vi "sonde front panel.vi"() -> ()   [LabVIEW 2016]
uses:
  SDI-12/Sonde Vertical Graph.ctl
  Waterloo DAQ/controls/Vertical Chart.ctl
  activeXtest/activeXtest 2015 Folder/sample data row cluster.ctl
  activeXtest/activeXtest 2015 Folder/sonde cluster.ctl
  Groundwater header.ctl
  Waterloo DAQ/controls/MCC DAQ Setup.ctl
  Waterloo DAQ/controls/Aux Sensor.ctl
  KPRO_2016 subvis/Control 2.ctl
  KPRO_2016 subvis/Control 9.ctl
  KPRO_2016 subvis/Graph Controls 2.ctl
  KPRO_2016 subvis/Ik control.ctl
  KPRO_2016 subvis/Ion Slope Control 8.ctl
  KPRO_2016 subvis/Depth Control.ctl
  KPRO_2016 subvis/SS Control 7.ctl
  Waterloo DAQ/controls/Action Control 1.ctl
  <extravilib>/ChannelInstances/One Element Stream-t'Action Control 1.ctl'/Instantiate.vi
  <extravilib>/ChannelInstances/One Element Stream-t'Action Control 1.ctl'/Endpoint.vi
  <vilib>/ULx/Create Channel.llb/ULx Create Channel (AI-Voltage-Basic).vi
  <vilib>/ULx/Read.llb/ULx Read (Analog DBL 1Chan 1Samp).vi
  C:/Program Files (x86)/National Instruments/LabVIEW 2016/vi.lib/ULx/ULx_LV.dll
  <vilib>/Utility/NIReport.llb/NI_report.lvclass
  <vilib>/Utility/config.llb/NI_LVConfig.lvlib
  <extravilib>/ChannelInstances/One Element Stream-t'Action Control 1.ctl'.lvlib
panel:
  out "Feet of Stainless 2":i32
  out "Feet of\nStainless to be\nUsed (Count)":i32
  in  "SS In":i32
  in  "Record Continuous Samples":bool
  out "Current Time (s)":dbl
  in  "Sample Sheet Data Row Cluster 2":T1={"Head"=0.0, "Depth"=0.0, "comment string"="", "Sonde Data Cluster"={"Cumulative\nVolume"=100.0, "Specific\nConductance"=2.0, "Dissolved\nOxygen"=3.0, "pH"=4.0, "ORP"=5.0, "Temp"=26.0, "Salinity"=7.0}} {"Sonde Data Cluster"."Salinity" format="%_3g"; "Sonde Data Cluster"."Temp" format="%_2g"; "Sonde Data Cluster"."ORP" format="%_4g"; "Sonde Data Cluster"."pH" format="%_4g"; "Sonde Data Cluster"."Dissolved\nOxygen" format="%_4g"; "Sonde Data Cluster"."Specific\nConductance" format="%_4g"; "Sonde Data Cluster"."Cumulative\nVolume" format="%#_4g"}
  in  "stop":bool
  in  "Write Data to Spreadsheet":bool
  in  "Sample Not Collected":bool
  in  "Record Single Sample":bool
  in  "Tab Control":T3(tab)
  out "12V Voltage Monitor":dbl format="%_3f"
  out "Found Quanta Sonde Com Port":refnum<visa-resource-name>
  in  "Temporary Data Files Directory":path=path "D:/Cascade/Data/Raw Sonde Data"
  in  "Data File Directory":path=path "D:/Cascade/Data/Excel Reports"
  out "Quanta Sonde found?":bool
  in  "report file path":path=path "D:/Cascade/templates/Groundwater Profiling Log_empty_2.xlsx"
  in  "template file path":path=path "D:/Cascade/templates/Groundwater Profiling Log_empty_labview_template.xlsx"
  in  "Config File Path":path=path "D:/Cascade/Data/config files/DAQ Setup Config.ini"
  in  "Read Configuration File?":bool=TRUE
  out "H-4191 Adapter found":bool
  in  "Save Configuration File?":bool
  out "Sonde Communication Error Out":errorcluster
  in  "Search for Comm Ports?":bool=TRUE
  in  "USB Serial Port Manual Entry":refnum<visa-resource-name>="COM13"
  in  "MCC USB-DAQ Setup":T4={"Device Name in InstaCal"="Dev0", "Omega Pressure Sensor"={"DAQ Channel"=2.0, "Output Voltage Range"=1, "Enabled"=TRUE, "Description"="Uphole Pressure"}, "McMillian 102 Flowmeter"={"DAQ Channel"=11.0, "Output Voltage Range"=1, "Enabled"=TRUE, "Description"="Flow"}, "DHT Pressure Sensor"={"DAQ Channel"=3.0, "Output Voltage Range"=1, "Enabled"=TRUE, "Description"="Downhole Pressure"}, "Top String Pot"={"DAQ Channel"=0.0, "Output Voltage Range"=0, "Enabled"=TRUE, "Description"="Top String Pot"}, "String Pot Signal"={"DAQ Channel"=1.0, "Output Voltage Range"=0, "Enabled"=TRUE, "Description"="String Pot"}, "Aux Sensor 1"={"DAQ Channel"=5.0, "Output Voltage Range"=1, "Enabled"=FALSE, "Description"="Aux 1"}, "Aux Sensor 2"={"DAQ Channel"=6.0, "Output Voltage Range"=1, "Enabled"=FALSE, "Description"="Aux 2"}, "Aux Sensor 3"={"DAQ Channel"=7.0, "Output Voltage Range"=1, "Enabled"=TRUE, "Description"="Aux 3"}, "Voltage Monitor"={"DAQ Channel"=8.0, "Output Voltage Range"=0, "Enabled"=TRUE, "Description"="9V Monitor"}} {"Voltage Monitor"."Output Voltage Range" items=["+/-10 V Range", "+/-5 V Range", "+/-2.5V Range", "+/-1.25 V Range", "+/-0.625 V Range", "+/-0.3125 V Range", "+/-0.1562V Range", "+/-0.078125 V Range"]; "Aux Sensor 3"."Output Voltage Range" items=["+/-10 V Range", "+/-5 V Range", "+/-2.5V Range", "+/-1.25 V Range", "+/-0.625 V Range", "+/-0.3125 V Range", "+/-0.1562V Range", "+/-0.078125 V Range"]; "Aux Sensor 2"."Output Voltage Range" items=["+/-10 V Range", "+/-5 V Range", "+/-2.5V Range", "+/-1.25 V Range", "+/-0.625 V Range", "+/-0.3125 V Range", "+/-0.1562V Range", "+/-0.078125 V Range"]; "Aux Sensor 1"."Output Voltage Range" items=["+/-10 V Range", "+/-5 V Range", "+/-2.5V Range", "+/-1.25 V Range", "+/-0.625 V Range", "+/-0.3125 V Range", "+/-0.1562V Range", "+/-0.078125 V Range"]; "String Pot Signal"."Output Voltage Range" items=["+/-10 V Range", "+/-5 V Range", "+/-2.5V Range", "+/-1.25 V Range", "+/-0.625 V Range", "+/-0.3125 V Range", "+/-0.1562V Range", "+/-0.078125 V Range"]; "Top String Pot"."Output Voltage Range" items=["+/-10 V Range", "+/-5 V Range", "+/-2.5V Range", "+/-1.25 V Range", "+/-0.625 V Range", "+/-0.3125 V Range", "+/-0.1562V Range", "+/-0.078125 V Range"]; "DHT Pressure Sensor"."Output Voltage Range" items=["+/-10 V Range", "+/-5 V Range", "+/-2.5V Range", "+/-1.25 V Range", "+/-0.625 V Range", "+/-0.3125 V Range", "+/-0.1562V Range", "+/-0.078125 V Range"]; "McMillian 102 Flowmeter"."Output Voltage Range" items=["+/-10 V Range", "+/-5 V Range", "+/-2.5V Range", "+/-1.25 V Range", "+/-0.625 V Range", "+/-0.3125 V Range", "+/-0.1562V Range", "+/-0.078125 V Range"]; "Omega Pressure Sensor"."Output Voltage Range" items=["+/-10 V Range", "+/-5 V Range", "+/-2.5V Range", "+/-1.25 V Range", "+/-0.625 V Range", "+/-0.3125 V Range", "+/-0.1562V Range", "+/-0.078125 V Range"]}
  out "Rate":dbl=1000.0 caption="Sample Rate (Hz)"
  out "Number of Channels":u16
  in  "Channel Data Rate S/s":dbl=3720.0 format="%#_13g"
  out "Descriptions":string[](array[string])
  out "Raw Voltages":dbl[](array[numeric])
  out "9V Voltage Monitor":dbl
  in  "Record DAQ Raw Voltages":bool
  in  "Groundwater Header":T6
  out "Worksheet Names":string[](array[string])
  in  "Current Sheet":i32=1
  out "row max value":i32
  out "last occupied cell's name":string
  out "Current Sample Sheet":string="Sample 1"
  in  "Cluster":T7={"Profile ID"="WP-01", "Hole Id"="HOLE_001"}
  out "Sonde Data Array":string[][](array[string])
  out "Table Label":string="Data from Sample Sheet %d from Excel File"
  out "Sonde Data Display":T8
  out "Temperature":cluster{"Y":dbl[], "Y":dbl[]}[](graph)
  in  "Record Reason":bool
  in  "Select Reasons to Record Data":u16(ring) items=["Per Client Request", "Timed Out", "Sample stopped flowing", "Equipment Issue"]
  in  "Record Calibration Values":bool
  in  "Ion Offset":dbl format="%.2f"
  in  "Ion Slope":dbl=44.04 format="%.2f"
  in  "Pressure \nSlope":dbl=24.27199935913086 format="%.2f"
  in  "Flow Slope":dbl=37.99800109863281 format="%.2f"
  in  "String Pot \nSlope":dbl=1.7339999675750732 format="%.2f"
  out "Slug Test\nIndicator copy":bool
  out "KPRO Test\nIndicator":bool
  in  "Start\nST":bool
  in  "Finish Tests":bool
  in  "Start  KPRO":bool
  in  "Feet of Stainless":i32=40
  out "Cluster 7":T10={"Flow"=0.21081600494384767, "Zeroed \nPressure"=74.74207969932556, "Ik"=0.003788962123473114, "Current Depth"=-100.6, "Feet of Stainless"=40, "Start Depth"=0.0, "Hole_Name_Path"=path "C:/e"} {"Start Depth" format="%.2f"; "Current Depth" format="%.2f"; "Ik" format="%.2f"; "Zeroed \nPressure" format="%.2f"; "Flow" format="%.2f"}
  in  "Cluster 2":T11={"Ion Slope"=44.04, "Ion Offset"=0.0, "Height of Sample Box"=0.0, "Last_Pressure_Slope"=48.27000045776367, "Last_Flow_Slope"=39.040000915527344, "Last_String_Pot_Slope"=1.6619999408721924} {"Last_String_Pot_Slope" format="%.2f"; "Last_Flow_Slope" format="%.2f"; "Last_Pressure_Slope" format="%.2f"; "Height of Sample Box" format="%.2f"; "Ion Offset" format="%.2f"; "Ion Slope" format="%.2f"}
  in  "Slope Cluster":T12={"Total Volume"=0.0, "String Pot Slope"=1.6619999408721924, "Flow Slope"=39.040000915527344, "Pressure Slope"=48.27000045776367, "Depth to Water Table"=-0.0, "Atmospheric Pressure"=32.22022530555725, "Reservoir Pressure"=-0.004827000045779073} {"Reservoir Pressure" format="%.2f"; "Atmospheric Pressure" format="%.2f"; "Depth to Water Table" format="%.2f"; "Pressure Slope" format="%.2f"; "Flow Slope" format="%.2f"; "String Pot Slope" format="%.2f"; "Total Volume" format="%.2f"}
  in  "Cluster 6":T13
  out "Cluster 4":T14={"Real Time - Depth vs. lk "={[0.003788962123473114, 0.0037174584307500765, 0.0037174584307500765, 0.0037174584307500765, 0.0037174584307500765, 0.003788962123473114], [-100.1, -100.2, -100.3, -100.4, -100.5, -100.6]}, "Real Time - Depth vs. lk  2"={[0.003788962123473114, 0.0037174584307500765, 0.0037174584307500765, 0.0037174584307500765, 0.0037174584307500765, 0.003788962123473114], [-100.1, -100.2, -100.3, -100.4, -100.5, -100.6]}, "Real Time - Depth vs. lk  2"={[0.003788962123473114, 0.0037174584307500765, 0.0037174584307500765, 0.0037174584307500765, 0.0037174584307500765, 0.003788962123473114], [-100.1, -100.2, -100.3, -100.4, -100.5, -100.6]}, "Ik "=0.003788962123473114, "Current Depth"=-100.6} {"Current Depth" format="%.2f"; "Ik" format="%.2f"}
  in  "Cluster 3":T15={"Cumulative - Depth vs. Ik"={[], []}, "Real Time - Depth vs. lk "={[0.003788962123473114, 0.0037174584307500765, 0.0037174584307500765, 0.0037174584307500765, 0.0037174584307500765, 0.003788962123473114], [-100.1, -100.2, -100.3, -100.4, -100.5, -100.6]}, "Cumulative - Depth vs. Drive"={[], []}, "Real Time - Depth vs. Drive"={[0.02036245163917736, 0.125, 0.16666666666666674, 0.16666666666666663, 0.16666666666666663, 0.16666666666666663], [-100.1, -100.2, -100.3, -100.4, -100.5, -100.6]}}
  out "DAQ Error":errorcluster
  out "Initialization Finished":bool=TRUE
  out "Stop":bool
  out "error out":errorcluster
  in  "error in (no error)":errorcluster
  out "producer loop":i32
  out "consumer loop":i32
  out "Active Channel Array":string[](array[string])
  out "delimited string":string
  out "Voltage Range":dbl[](array[numeric])
  out "Stop 2":bool
  # "Instructions for Sonde Calibration:\n1.  Use the Record Single Point to Record the Data for the specific parameter.\n2."
  # "String Pot"
  # "Use Incr"
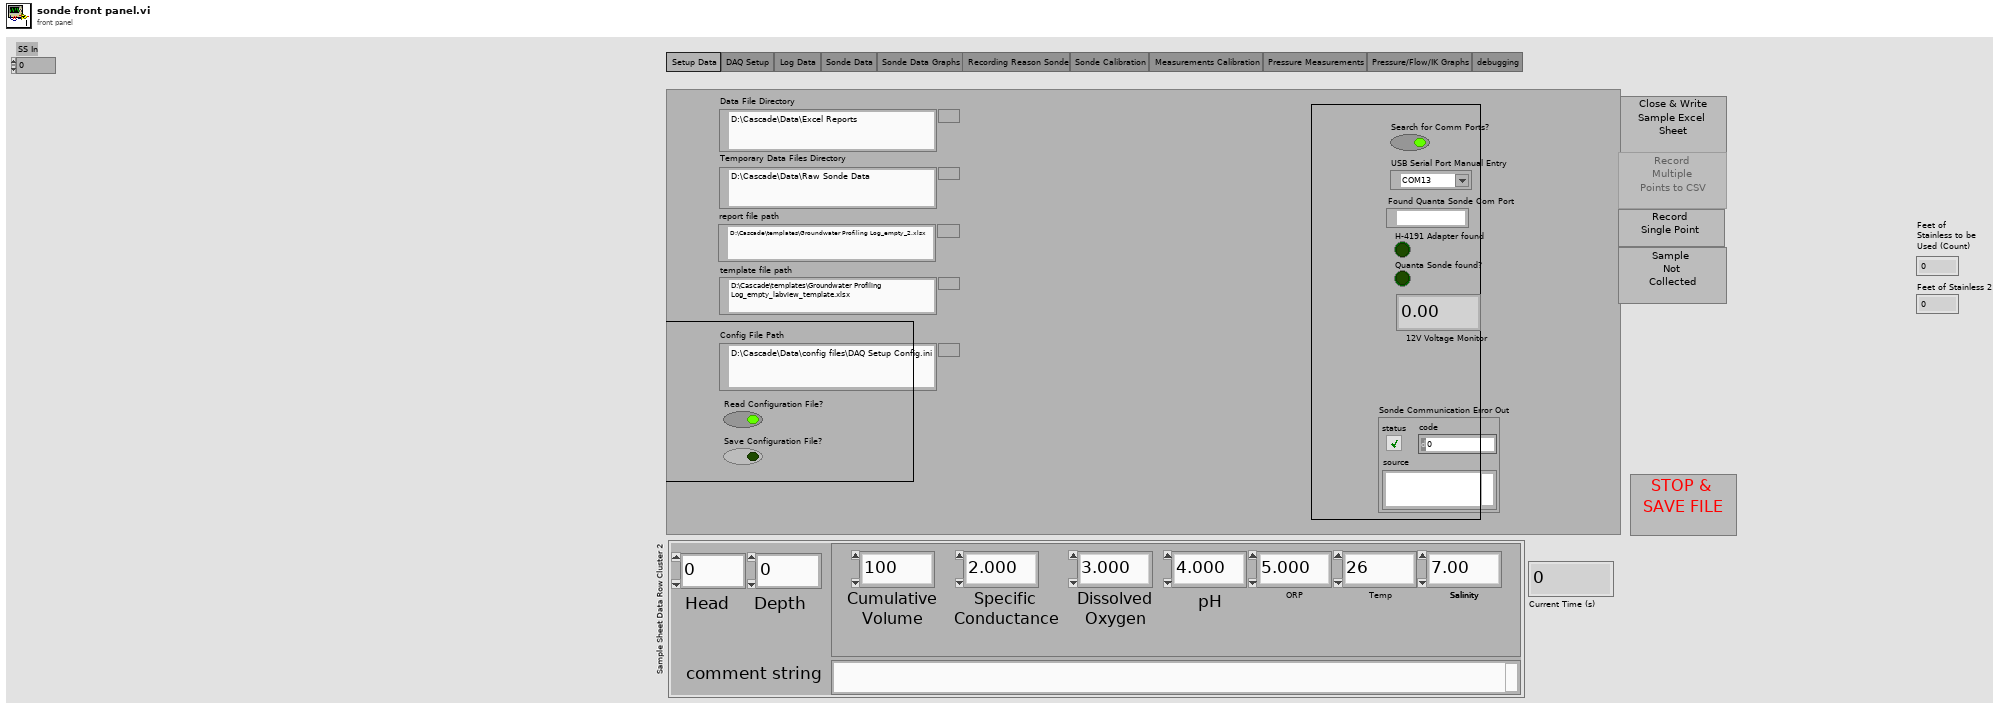
[diagram p1: front panel]
types:
  T1 = typedef "sample data row cluster.ctl" = cluster{"Head":dbl, "Depth":dbl, "comment string":string, "Sonde Data Cluster":T2}
  T2 = typedef "sonde cluster.ctl" = cluster{"Cumulative\nVolume":dbl, "Specific\nConductance":dbl, "Dissolved\nOxygen":dbl, "pH":dbl, "ORP":dbl, "Temp":dbl, "Salinity":dbl}
  T3 = enum32{"Setup Data", "DAQ Setup", "Log Data", "Sonde Data", "Sonde Data Graphs", "Recording Reason Sonde", "Sonde Calibration", "Measurements Calibration", "Pressure Measurements", "Pressure/Flow/IK Graphs", "debugging"}
  T4 = typedef "MCC DAQ Setup.ctl" = cluster{"Device Name in InstaCal":string, "Omega Pressure Sensor":T5, "McMillian 102 Flowmeter":T5, "DHT Pressure Sensor":T5, "Top String Pot":T5, "String Pot Signal":T5, "Aux Sensor 1":T5, "Aux Sensor 2":T5, "Aux Sensor 3":T5, "Voltage Monitor":T5}
  T5 = typedef "Aux Sensor.ctl" = cluster{"DAQ Channel":dbl, "Output Voltage Range":u16, "Enabled":bool, "Description":string}
  T6 = typedef "Groundwater header.ctl" = cluster{"Location":string, "Date Finished":string, "CTS":string, "sampler":string, "Kpro box Serial ":string, "Sonde Serial":string, "Drilling Contractor":string, "Ave Depth to Water":string, "Gas/Peri Pump":string, "Atmospheric Pressure":string, "KPRO N2 Pressure":string, "Gas Drive N2 Pressure":string}
  T7 = typedef "Control 9.ctl" = cluster{"Profile ID":string, "Hole Id":string}
  T8 = typedef "Sonde Vertical Graph.ctl" = cluster{"pH":T9, "Conductance":T9, "Salinity":T9, "DO % Saturation":T9, "DO mg/L":T9, "ORP":T9}
  T9 = typedef "Vertical Chart.ctl" = cluster{"Y":dbl[], "Y":dbl[]}[]
  T10 = typedef "SS Control 7.ctl" = cluster{"Flow":dbl, "Zeroed \nPressure":dbl, "Ik":dbl, "Current Depth":sgl, "Feet of Stainless":i32, "Start Depth":sgl, "Hole_Name_Path":path}
  T11 = typedef "Ion Slope Control 8.ctl" = cluster{"Ion Slope":dbl, "Ion Offset":dbl, "Height of Sample Box":dbl, "Last_Pressure_Slope":dbl, "Last_Flow_Slope":dbl, "Last_String_Pot_Slope":dbl}
  T12 = typedef "Control 2.ctl" = cluster{"Total Volume":dbl, "String Pot Slope":dbl, "Flow Slope":dbl, "Pressure Slope":dbl, "Depth to Water Table":dbl, "Atmospheric Pressure":dbl, "Reservoir Pressure":dbl}
  T13 = typedef "Depth Control.ctl" = cluster{"Depth mode":bool, "Increment\nButton":bool}
  T14 = typedef "Ik control.ctl" = cluster{"Real Time - Depth vs. lk ":cluster{dbl[], dbl[]}, "Real Time - Depth vs. lk  2":cluster{dbl[], dbl[]}, "Real Time - Depth vs. lk  2":cluster{dbl[], dbl[]}, "Ik ":dbl, "Current Depth":sgl}
  T15 = typedef "Graph Controls 2.ctl" = cluster{"Cumulative - Depth vs. Ik":cluster{dbl[], dbl[]}, "Real Time - Depth vs. lk ":cluster{dbl[], dbl[]}, "Cumulative - Depth vs. Drive":cluster{dbl[], dbl[]}, "Real Time - Depth vs. Drive":cluster{dbl[], dbl[]}}
  T16 = typedef "Action Control 1.ctl" = enum16{"TimeOut", "Continuous  Data", "Init", "Exit", "Acq. Single Point", "Write Sample Sheet", "Acq. DAQ data", "Sample Not Collected", "Record Reason"}
  T17 = typedef "NI_LVConfig.lvlib/Config Data RefNum.ctl" = refnum<k1>
  T18 = enum8{"Enabled", "Disabled", "Disabled and Grayed Out"}
  T19 = typedef "One Element Stream-t'Action Control 1.ctl'.lvlib/)Channel.ctl" = refnum<queue>
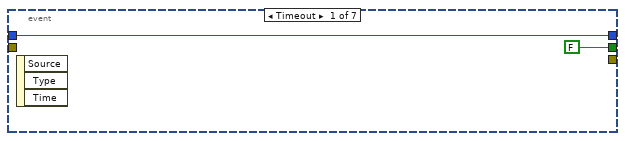
[diagram p2: hidden frame]
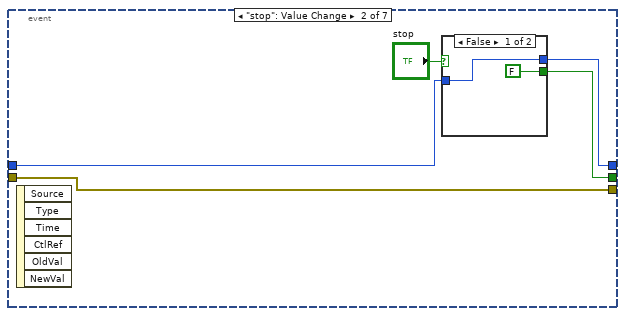
[diagram p3: hidden frame]
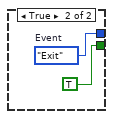
[diagram p4: hidden frame]
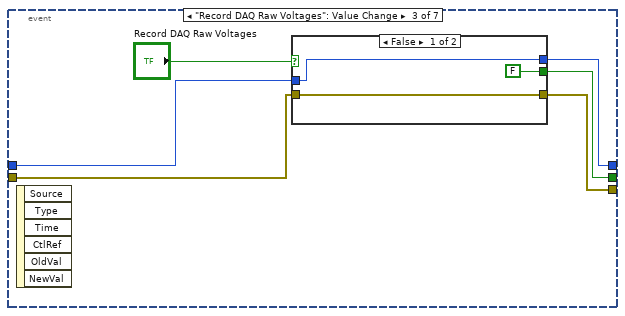
[diagram p5: hidden frame]
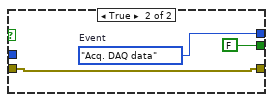
[diagram p6: hidden frame]
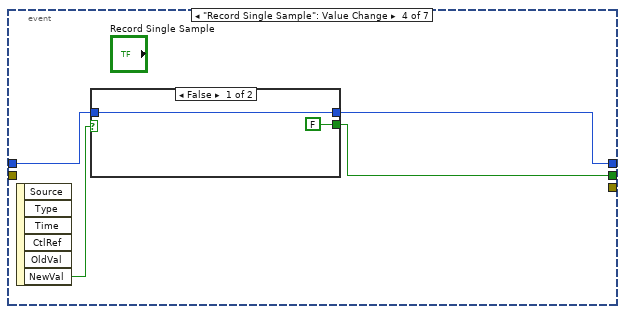
[diagram p7: hidden frame]
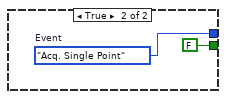
[diagram p8: hidden frame]
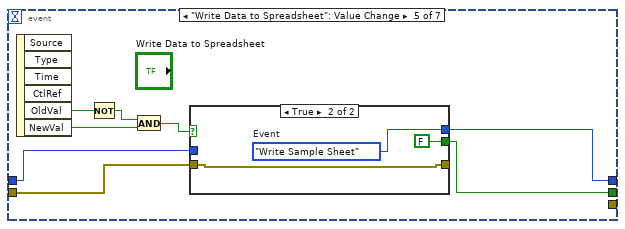
[diagram p9: hidden frame]
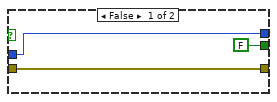
[diagram p10: hidden frame]
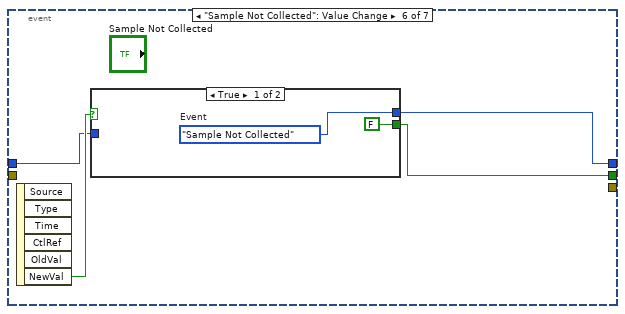
[diagram p11: hidden frame]
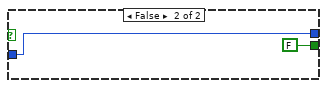
[diagram p12: hidden frame]
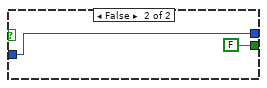
[diagram p13: hidden frame]
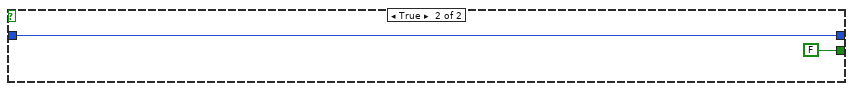
[diagram p14: hidden frame]
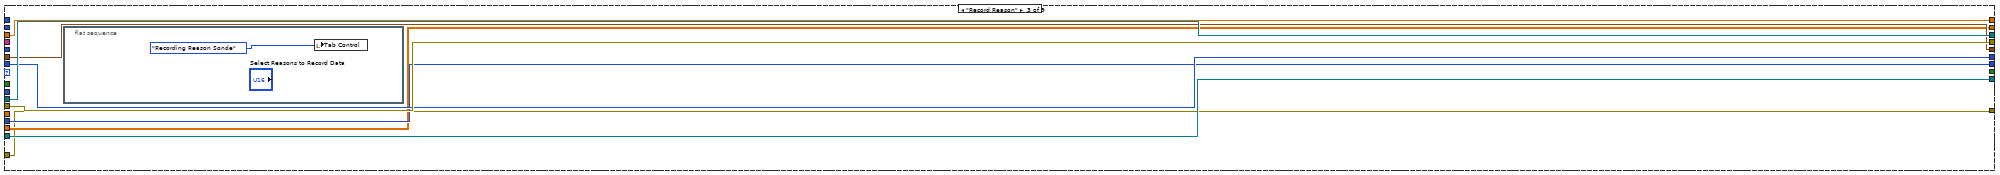
[diagram p16: hidden frame]
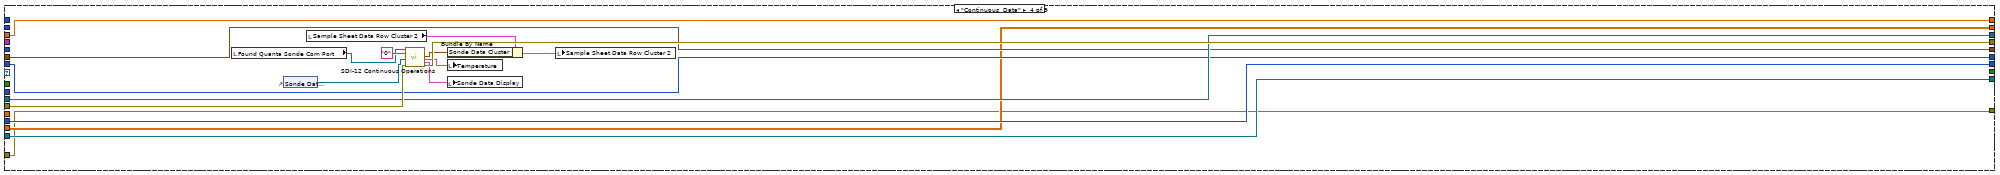
[diagram p17: hidden frame]
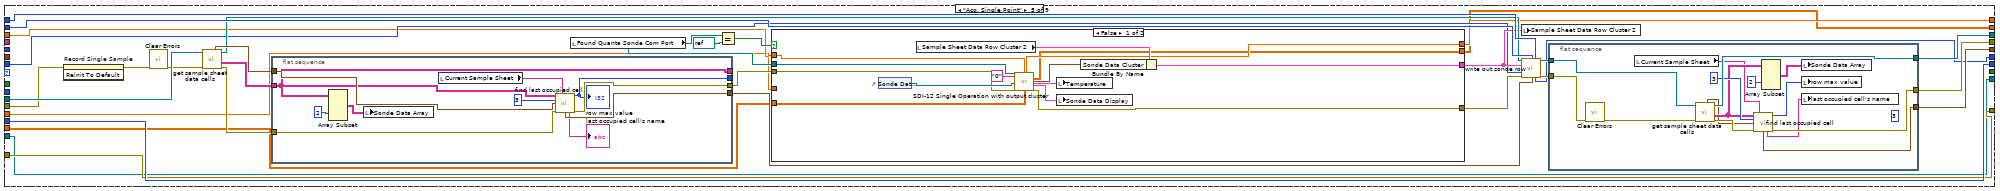
[diagram p18: hidden frame]
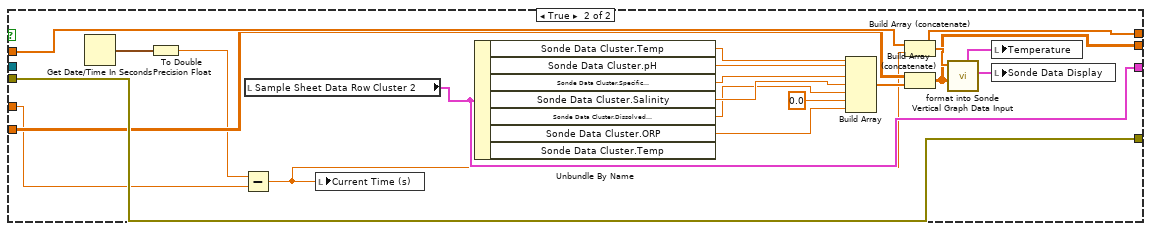
[diagram p19: hidden frame]
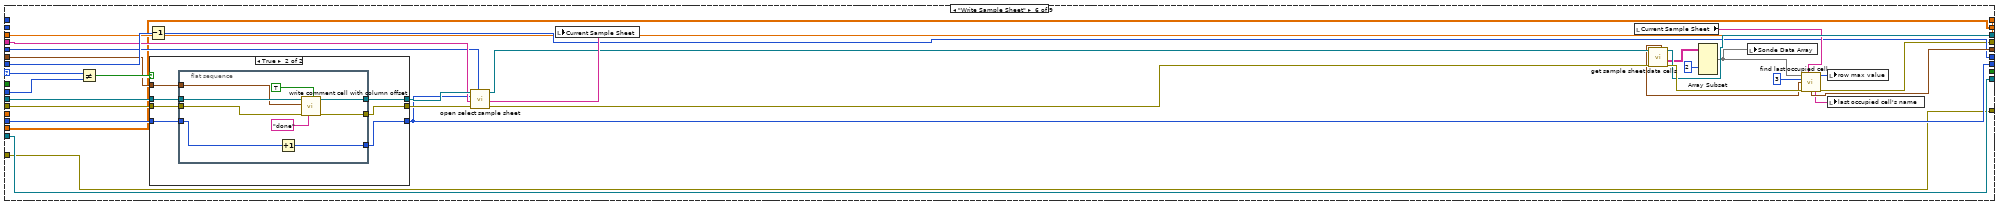
[diagram p20: hidden frame]
diagram:
  w7 = Action_Control_1."Init"  # Event
  # "For calibrate command (XC) on SDI-12 address ‘a’, P is pH, C is specific conductance, S is\nsalinity or TDS, % is DO %Saturation, O is DO mg/L, R is ORP, D is depth, B is\nbarometric pressure, and t is TDS scale factor."
  n1 = flat-sequence {
    tunnel: [w31] -> w10
    tunnel: [w63] -> w16
    tunnel: w10 -> [w63]
    tunnel: [w59] -> w6
    tunnel: [w74] -> w26
    tunnel: w16 -> [w71]
    tunnel: [w71] -> w11
    tunnel: w26 -> [w130]
    tunnel: [w102] -> w24
    tunnel: [w106] -> w22
    tunnel: [w113] -> w17
    tunnel: [w112] -> w19
    tunnel: [w111] -> w20
    tunnel: [w104] -> _
    tunnel: [w100] -> w25
    tunnel: ["Feet of Stainless"] -> w5
    tunnel: [w97] -> w4
    tunnel: [w96] -> w3
    frame #0 {
      n2 = flat-sequence {
        tunnel: [w35] -> w31
        tunnel: "error in (no error)" -> [w34]
        frame #0 {
          n3 = case shown="False" "Read Configuration File?" {
            selector: "Read Configuration File?" -> [_ w42]
            tunnel: [w36 w47] -> w35
            tunnel: w34 -> [w36 w44]
            tunnel: "Config File Path" -> [_ w43]
            frame False {
            }
            frame True {
              n4 = call <vilib>:"Check if File or Folder Exists.vi"("error in (no error)"=w44, "path"=w43) -> ("error out"=w39:errorcluster, "file or folder exists?"=w40:bool, "dup path"=w38:path)  [unwired: 7 in]
              n5 = And(x=w42, y=w40) -> (x .and. y?=w41:bool)
              n6 = control-ref of="This VI"() -> (w45:refnum<vi>)
              n7 = case shown="True" w41 {
                selector: w41 -> [w48 _]
                tunnel: w38 -> [_ w53]
                tunnel: w39 -> [w49 w57]
                tunnel: [w49 w50] -> w46
                tunnel: w45 -> [_ w58]
                frame False {
                  n8 = local write "Read Configuration File?"(w48) -> ()
                }
                frame True {
                  n9 = call <vilib>:"Open Config Data.vi"("error in (no error)"=w57, "create file if necessary (T)"=FALSE, "configuration file path"=w53) -> ("error out"=w55:errorcluster, "refnum"=w56:T17)  [unwired: 6 in, 1 out]
                  n10 = call <userlib>:"Read Panel from INI__ogtk.vi"("error in (no error)"=w55, "VI ref"=w58, "refnum"=w56) -> ("error out"=w51:errorcluster, "refnum out"=w52:T17)  [unwired: 7 in]
                  n11 = call <vilib>:"Close Config Data.vi"("error in (no error)"=w51, "refnum"=w52) -> ("error out"=w50:errorcluster)  [unwired: 8 in, 1 out]
                }
              }
              n12 = call <vilib>:"Clear Errors.vi"("error in (no error)"=w46) -> ("error out"=w37:errorcluster)  [unwired: 5 in, 1 out]
              n13 = Merge Errors(w37) -> (w47:errorcluster)
            }
          }
        }
      }
      n14 = invoke on="error out" class="Clust (strict)" method="Reinit To Default"(error in="error in (no error)") -> ()  [unwired: 2 in, 3 out]
    }
    frame #1 {
      n15 = Get Date/Time In Seconds() -> (seconds since 1Jan1904=w60:timestamp)
      n16 = Get Date/Time In Seconds() -> (seconds since 1Jan1904=w59:timestamp)
      n17 = local write "Current Sheet"(1 ("Current Sheet")) -> ()
      n18 = Subtract(x=w59, y=w60) -> (x-y=w61:dbl)
      n19 = To Double Precision Float(number=w61) -> (double precision float=→"Current Time (s)":dbl)
    }
    frame #2 {
      w83 = T18."Disabled and Grayed Out" ("Disabled")
      (unwired) FALSE ("Stop")
      n20 = control-ref of="Sonde Data Display"() -> ()  [unwired: 1 out]
      n21 = invoke on="Current Sheet" class="DigNum (strict)" method="Reinit To Default"() -> (error out=w76:errorcluster)  [unwired: 3 in, 2 out]
      n22 = local write "Initialization Finished"(FALSE ("Initialization Finished")) -> ()
      n23 = local write "Groundwater Header"(T6 {"Location"="Randolph VT", "Date Finished"="", "CTS"="123456789", "sampler"="MM", "Kpro box Serial "="12345", "Sonde Serial"="Quanta ", "Drilling Contractor"="ARA", "Ave Depth to Water"="0.00", "Gas/Peri Pump"="Peri", "Atmospheric Pressure"="760mm", "KPRO N2 Pressure"="69.35psi", "Gas Drive N2 Pressure"="NA"} ("Groundwater Header 2")) -> ()
      n24 = invoke on="Sample Not Collected" class="Bool" method="Reinit To Default"(error in=w76) -> (error out=w80:errorcluster)  [unwired: 2 in, 2 out]
      n25 = invoke on="Record Continuous Samples" class="Bool" method="Reinit To Default"(error in=w80) -> (error out=w79:errorcluster)  [unwired: 2 in, 2 out]
      n26 = property on="Record Continuous Samples" class="Bool"("DisabledEnum"=w83) -> (error out=w84:errorcluster)  [unwired: 2 in, 1 out]
      n27 = call "search for Quanta Sonde devices.vi"("VISA resource name"="USB Serial Port Manual Entry", "Search for Comm Ports?"="Search for Comm Ports?", "error in (no error)"=w71) -> ("12V monitor"=→"12V Voltage Monitor":dbl, "Com Port with Quanta Sonde devices"=w90:refnum<visa-resource-name>[], "Number of Quanta Sonde devices"=w89:i32, "Number of Quanta Sonde devices > 0?"=→"Quanta Sonde found?":bool, "H-4191 Adapter found"=→"H-4191 Adapter found":bool, "Error Out"=w68:errorcluster)  [unwired: 5 in, 2 out]
      "Sonde Communication Error Out" <- w68
      n28 = case shown="0, Default" w89 {
        tunnel: w90 -> [_ w95]
        tunnel: [refnum<visa-resource-name> refnum ("RS232 Port Out") w93] -> w88
        frame 0, Default {
        }
        frame 1 {
          n29 = Index Array(array=w95, index=0) -> (element=w93:refnum<visa-resource-name>)
        }
      }
      "Found Quanta Sonde Com Port" <- w88
      n30 = invoke on="Write Data to Spreadsheet" class="Bool" method="Reinit To Default"(error in=w79) -> (error out=w78:errorcluster)  [unwired: 2 in, 2 out]
      n31 = property on="Record Single Sample" class="Bool"(error in=w84, "DisabledEnum"=w83) -> (error out=w85:errorcluster)  [unwired: 1 in, 1 out]
      n32 = invoke on="Record Single Sample" class="Bool" method="Reinit To Default"(error in=w78) -> (error out=w77:errorcluster)  [unwired: 2 in, 2 out]
      n33 = call <vilib>:"Clear Errors.vi"("error in (no error)"=w68) -> ("error out"=w67:errorcluster)  [unwired: 5 in, 1 out]
      n34 = invoke on="stop" class="Bool" method="Reinit To Default"(error in=w77) -> (error out=w82:errorcluster)  [unwired: 2 in, 2 out]
      n35 = invoke on="Stop" class="Bool (strict)" method="Reinit To Default"() -> (error out=w70:errorcluster)  [unwired: 3 in, 2 out]
      n36 = property on="Write Data to Spreadsheet" class="Bool"(error in=w82, "DisabledEnum"=w83) -> (error out=w73:errorcluster)  [unwired: 1 in, 1 out]
      n37 = property on="Sample Not Collected" class="Bool"(error in=w85, "DisabledEnum"=w83) -> (error out=w81:errorcluster)  [unwired: 1 in, 1 out]
      n38 = invoke on="Stop 2" class="Bool (strict)" method="Reinit To Default"(error in=w70) -> (error out=w69:errorcluster)  [unwired: 2 in, 2 out]
      n39 = Merge Errors(w67, w69, w73, w81) -> (w74:errorcluster)
    }
    frame #3 {
      w105 = "Sample 1" ("Worksheet Name in")
      n40 = flat-sequence {
        frame #0 {
        }
      }
      n41 = call "get sample header columns.vi"("error in (no error)"=w130) -> ("Column of Volume"=w112:i32, "Columns"=w111:i32[], "data"=w123:string[][], "error out"=w131:errorcluster)  [unwired: 5 in, 6 out]
      n42 = call "close excel file if open.vi"("error in (no error)"=w131, "report file path in"="report file path") -> ("error out"=w116:errorcluster, "report file path out"=w99:path)  [unwired: 8 in]
      n43 = Index Array(array=w123, index (col)=0 ("disabled index (col)")) -> (element=w122:string[])  [unwired: 1 in]
      n44 = flat-sequence {
        tunnel: [w132] -> w96
        frame #0 {
          n45 = Unbundle By Name("Slope Cluster") -> ("Depth to Water Table"=w135:dbl)
          n46 = call "New Stainless Correction Pop Up 2016.vi"("New Feet\n of Stainless\n(Count)"="SS In", "Depth to \nWater Table\nInput"=w135) -> ("Feet of\nStainless to be\nUsed (Count)"=w132:i32, "Depth to \nWater Table\nOutput"=w133:dbl)  [unwired: 2 in]
          n47 = Bundle By Name(cluster="Slope Cluster", "Depth to Water Table"=w133) -> (w136:T12)
          n48 = local write "Slope Cluster"(w136) -> ()
        }
      }
      n49 = call "copy excel template.vi"("error in (no error)"=w116, "report file path in"=w99, "template file path in"="template file path") -> ("error out"=w117:errorcluster, "report file path out"=w119:path)  [unwired: 7 in]
      n50 = Array Size(array=w122) -> (size(s)=w129:i32)
      n51 = Initialize Array("", 10 ("dimension size"), w129) -> (w127:string[][])
      n52 = call "open excel get worksheet names.vi"("error in (no error)"=w117, "milliseconds to wait"=u32 5, "report file path"=w119) -> ("error out"=w114:errorcluster, "Number of Sample Sheets"=w113:i32, "NI_report out"=w115:refnum<class "NI_report.lvclass">, "Worksheet Names"=w106:string[])  [unwired: 3 in, 2 out]
      "Worksheet Names" <- w106
      n53 = flat-sequence {
        tunnel: w114 -> [w160]
        tunnel: [w159] -> w108
        tunnel: [w156] -> w109
        tunnel: [w158] -> _
        tunnel: w106 -> [w157]
        tunnel: w115 -> [w156]
        frame #0 {
          n54 = call "groundwater log header.vi"("Worksheet Names"=w157, "Groundwater Header"="Groundwater Header", "error in (no error)"=w160, "NI_report in"=w156) -> ("error out"=w159:errorcluster, "NI_report out"=w158:refnum<class "NI_report.lvclass">)  [unwired: 6 in]
        }
      }
      n55 = Insert Into Array(array=w127, index (row)=0, new element=w122) -> (→"Sonde Data Array":string[][])  [unwired: 1 in]
      n56 = flat-sequence {
        tunnel: [w138] -> w97
        frame #0 {
          # "KPRO Array"
          n57 = Initialize Array(0.0, 0, 9) -> (w138:dbl[][])
        }
      }
      n58 = local write "Current Sample Sheet"(w105) -> ()
      n59 = call "find and open select worksheet.vi"("Worksheet Names"=w106, "error in (no error)"=w108, "milliseconds to wait"=u32 100, "Worksheet Name in"=w105, "NI_report in"=w109) -> ("error out"=w101:errorcluster, "Select Worksheet Index"=w104:i32, "NI_report out"=w103:refnum<class "NI_report.lvclass">)  [unwired: 4 in]
      n60 = flat-sequence {
        tunnel: w101 -> [w155]
        tunnel: w103 -> [w154]
        tunnel: [w153] -> w102
        tunnel: [w147] -> w100
        tunnel: [w145] -> _
        frame #0 {
          (unwired) 3 ("Header Rows to remove")
          n61 = local read "Current Sample Sheet"() -> (w143:string)
          n62 = call "get sample sheet data cells.vi"("error in (no error)"=w155, "NI_report in"=w154) -> ("error out"=w148:errorcluster, "data"=w149:string[][], "NI_report out"=w153:refnum<class "NI_report.lvclass">, "left edge output cluster"=w146:cluster{"row":i32, "column":i32})  [unwired: 5 in, 1 out]
          n63 = call "find last occupied cell.vi"("data"=w149, "Active Sheet"=w143, "Header Rows to remove"=3, "sub array start"=w146, "error in (no error)"=w148) -> ("row max value"=w144:i32, 13:"start of last occupied row"=w145:cluster{"row":i32, "column":i32}, 14:"start of last occupied row"=w142:string, "error out"=w147:errorcluster)  [unwired: 4 in, 3 out]
          n64 = Array Subset(array=w149, index (col)=2 ("index")) -> (w151:string[][])  [unwired: 3 in]
          n65 = local write "Sonde Data Array"(w151) -> ()
          n66 = local write "row max value"(w144) -> ()
          n67 = local write "last occupied cell's name"(w142) -> ()
        }
      }
    }
  }
  n68 = while {
    shift-right: [w169] -> w29
    shift-left: w25 -> [w169]
    shift-right: [w164] -> _
    shift-left: w7 -> [w162]
    tunnel: [w170] -> w9
    i -> [w168]
    stop <- w166 stop-if-true
    # "User Interface Producer Loop"
    n69 = First Call?() -> (First Call?: T/F=w163:bool)
    n70 = case shown="False" w163 {
      tunnel: w169 -> [w175 _]
      tunnel: [w173 FALSE ("Boolean")] -> w166
      tunnel: [w172 w238] -> w164
      tunnel: w162 -> [_ w238]
      frame False {
        w171 = Action_Control_1."TimeOut"  # Event
        n71 = event shown="[6] \"Record Reason\": Value Change" {
          selector: _ -> [_ _ _ _ _ _ _]
          dyn-events: _ -> [_ _ _ _ _ _ _]
          timeout: 100 -> [_ _ _ _ _ _ _]
          tunnel: [w176 w182 w188 w202 w213 w223 w231] -> w172
          tunnel: [FALSE w181 w189 w201 w212 w224 w232] -> w173
          tunnel: w175 -> [_ w179 w191 _ w209 _ _]
          tunnel: [_ w179 w190 _ _ _ _] -> _
          tunnel: w171 -> [w176 w178 w187 w199 w207 w221 w229]
          event Timeout {
            n72 = event-data() -> ()  [unwired: 1 in, 3 out]
          }
          event "stop": Value Change {
            n73 = event-data() -> ()  [unwired: 1 in, 6 out]
            n74 = case shown="False" "stop" {
              tunnel: [w183 w185] -> w182
              tunnel: [FALSE TRUE] -> w181
              tunnel: w178 -> [w183 _]
              frame False {
              }
              frame True {
                w185 = Action_Control_1."Exit"  # Event
              }
            }
          }
          event "Record DAQ Raw Voltages": Value Change {
            n75 = event-data() -> ()  [unwired: 1 in, 6 out]
            n76 = case shown="False" "Record DAQ Raw Voltages" {
              tunnel: [w193 w196] -> w188
              tunnel: [FALSE FALSE ("Boolean")] -> w189
              tunnel: [w194 w197] -> w190
              tunnel: w191 -> [w194 w197]
              tunnel: w187 -> [w193 _]
              frame False {
              }
              frame True {
                w196 = Action_Control_1."Acq. DAQ data"  # Event
              }
            }
          }
          event "Record Single Sample": Value Change {
            n77 = event-data() -> ("NewVal"=w200:bool)  [unwired: 1 in, 5 out]
            n78 = case shown="False" w200 {
              tunnel: [w203 w205] -> w202
              tunnel: [FALSE FALSE] -> w201
              tunnel: w199 -> [w203 _]
              frame False {
              }
              frame True {
                w205 = Action_Control_1."Acq. Single Point"  # Event
              }
            }
          }
          event "Write Data to Spreadsheet": Value Change {
            n79 = event-data() -> ("OldVal"=w211:bool, "NewVal"=w214:bool)  [unwired: 1 in, 4 out]
            n80 = Not(x=w211) -> (.not. x?=w210:bool)
            n81 = And(x=w210, y=w214) -> (x .and. y?=w208:bool)
            n82 = case shown="True" w208 {
              tunnel: [w215 w218] -> w213
              tunnel: [FALSE FALSE ("Boolean")] -> w212
              tunnel: [w216 w219] -> _
              tunnel: w209 -> [w216 w219]
              tunnel: w207 -> [w215 _]
              frame False {
              }
              frame True {
                w218 = Action_Control_1."Write Sample Sheet"  # Event
              }
            }
          }
          event "Sample Not Collected": Value Change {
            n83 = event-data() -> ("NewVal"=w222:bool)  [unwired: 1 in, 5 out]
            n84 = case shown="True" w222 {
              tunnel: [FALSE FALSE] -> w224
              tunnel: [w225 w227] -> w223
              tunnel: w221 -> [_ w227]
              frame True {
                w225 = Action_Control_1."Sample Not Collected"  # Event
              }
              frame False {
              }
            }
          }
          event "Record Reason": Value Change {
            n85 = event-data() -> ("NewVal"=w230:bool)  [unwired: 1 in, 5 out]
            n86 = case shown="True" w230 {
              tunnel: [FALSE FALSE] -> w232
              tunnel: [w233 w235] -> w231
              tunnel: w229 -> [_ w235]
              frame True {
                w233 = Action_Control_1."Record Reason"  # Event
              }
              frame False {
              }
            }
          }
        }
      }
      frame True {
      }
    }
    "Stop" <- w166
    n87 = local read "Stop"() -> (w167:bool)
    n88 = Or(x=w167, y=w166) -> ()  [unwired: 1 out]
    n89 = call <extravilib>:"Write With Abort.vi"("abort"=FALSE, "last element? (F)"=w166, "element"=w164) -> ("channel"=w170:T19)  [unwired: 6 in, 2 out]
    "producer loop" <- w168
  }
  n90 = Get Date/Time In Seconds() -> (seconds since 1Jan1904=w13:timestamp)
  n91 = To Double Precision Float(number=w13) -> (double precision float=w12:dbl)
  n92 = while {
    tunnel: w25 -> [w274]
    tunnel: [w276] -> w28
    tunnel: w9 -> [w245]
    tunnel: w24 -> [w272]
    shift-right: [w260] -> _
    shift-left: "Current Sheet" -> [w266]
    tunnel: w22 -> [w262]
    tunnel: w20 -> [w270]
    tunnel: w19 -> [w269]
    shift-right: [w261] -> _
    shift-left: 0 ("row index") -> [w268]
    tunnel: [w267] -> _
    shift-right: [w265] -> _
    shift-left: cluster{"row":i32, "column":i32} {"row"=0, "column"=0} ("start of last occupied row") -> [w264]
    tunnel: w17 -> [w259]
    shift-right: [w253] -> _
    shift-left: dbl[] [] ("Time Array") -> [w254]
    shift-right: [w252] -> _
    shift-left: dbl[][] [] ("Time Array") -> [w251]
    tunnel: w12 -> [w250]
    tunnel: [w248] -> _
    tunnel: w11 -> [w247]
    shift-right: [w243] -> _
    shift-left: refnum<k24>[] [] -> [w249]
    tunnel: w6 -> [w241]
    shift-right: [w240] -> w1
    shift-left: w5 -> [w240]
    tunnel: w4 -> [_]
    shift-right: [w239] -> w2
    shift-left: w3 -> [w239]
    i -> [w275]
    stop <- w246 stop-if-true
    # "Consumer Data Handling Loop"
    n93 = call <extravilib>:"Read With Abort.vi"("abort"=FALSE, "channel"=w245) -> ("last element?"=w244:bool, "element"=w256:T16)  [unwired: 5 in, 3 out]
    n94 = call <userlib>:"Wait (ms)__ogtk.vi"("error in (no error)"=w274, "milliseconds to wait"=u32 50) -> ("error out"=w258:errorcluster)  [unwired: 8 in, 1 out]
    n95 = feedback-in #1(w256) -> ()
    n96 = feedback #1() -> (w255:T16)  [unwired: 1 in]
    n97 = flat-sequence {
      frame #0 {
        n98 = call "Get_SLOPE_data_from_file 2016.vi"() -> ()  [unwired: 8 in, 4 out]
        n99 = call "Pressure 2016.vi"() -> ()  [unwired: 3 in, 1 out]
        n100 = call "In-Line-Pressure 2016.vi"() -> ()  [unwired: 4 in, 1 out]
        n101 = call "boolean debounce 2016.vi"() -> ()  [unwired: 1 in, 1 out]
        n102 = call "Flow 2016.vi"() -> ()  [unwired: 3 in, 1 out]
      }
    }
    n103 = call "open select sample sheet.vi"("Number of Sample Sheets"=w259, "error in (no error)"=w258, "Worksheet Names"=w262, "Active Sample Sheet"=w266, "NI_report in"=w272) -> ("error out"=w273:errorcluster, "Current Sample Sheet"=w242:string, "NI_report out"=w271:refnum<class "NI_report.lvclass">)  [unwired: 3 in, 1 out]
    n104 = flat-sequence {
      tunnel: w242 -> [w282]
      tunnel: w241 -> [w277]
      frame #0 {
        n105 = Get Date/Time In Seconds() -> (seconds since 1Jan1904=w278:timestamp)
        n106 = Scan From String(format string="Sample %d", input string=w282) -> (output 1=w280:i32)  [unwired: 3 in, 3 out]
        n107 = Subtract(x=w278, y=w277) -> (x-y=w279:dbl)
        n108 = Format Into String(format string="Data from Sample Sheet %d from Excel File", w280) -> (resulting string=→"Table Label":string)  [unwired: 2 in, 1 out]
        n109 = local write "Current Time (s)"(w279) -> ()
        "Current Sample Sheet" <- w282
      }
    }
    n110 = case shown="\"Sample Not Collected\"" w256 {
      selector: w256 -> [_ _ _ _ _ w445 _ _ _]
      tunnel: w273 -> [w293 w303 w312 w329 w345 w454 w478 w528 w548]
      tunnel: [w293 w303 w312 w328 w343 w424 w478 w528 w540] -> w276
      tunnel: w244 -> [_ _ _ _ _ _ _ _ _]
      tunnel: w271 -> [w292 w302 w311 w321 w363 w456 w487 w527 w547]
      tunnel: [w291 w301 w310 w320 w340 w429 w486 w526 w545] -> w261
      tunnel: w270 -> [_ _ _ _ w358 _ _ _ _]
      tunnel: w269 -> [_ _ _ _ w357 _ _ _ _]
      tunnel: w268 -> [w291 w301 w310 w320 w341 w455 w486 w526 w545]
      tunnel: [w292 w302 w311 w321 w346 w450 w487 w527 w546] -> w267
      tunnel: w266 -> [w290 w300 w309 w319 w354 w447 w485 w525 w544]
      tunnel: [w290 w300 w309 w319 w354 w446 w485 w525 w544] -> w260
      tunnel: [w289 w299 w308 w318 w342 w441 w484 w524 w543] -> w265
      tunnel: w264 -> [w289 w299 w308 w318 _ w442 w484 w524 w543]
      tunnel: w262 -> [_ _ _ _ _ w449 _ _ _]
      tunnel: w259 -> [_ _ _ _ _ w448 _ _ _]
      tunnel: w255 -> [_ _ _ _ _ w444 _ _ _]
      tunnel: w254 -> [w288 w298 w307 w317 w339 w428 w483 w523 w542]
      tunnel: [w288 w298 w307 w317 w338 w428 w483 w523 w542] -> w253
      tunnel: [w287 w297 w306 w316 w337 w427 w482 w522 w541] -> w252
      tunnel: w251 -> [w287 w297 w306 w316 w336 w427 w482 w522 w541]
      tunnel: w250 -> [_ _ _ _ w335 _ _ _ _]
      tunnel: w249 -> [w286 w296 w305 w315 w333 w426 _ w520 w535]
      tunnel: [w285 w295 w304 w314 w334 w425 w476 _ w536] -> w248
      tunnel: w247 -> [w285 w295 w304 w314 w334 w425 w479 w519 w539]
      tunnel: [_ _ _ _ _ _ FALSE ("aborted?") FALSE ("aborted?") w538] -> w246
      tunnel: [w286 w296 w305 w315 w333 w426 w480 w517 w535] -> w243
      frame "TimeOut", Default {
      }
      frame "Sample Not Collected" {
        n111 = local write "Tab Control"(T3."Recording Reason Sonde" ("Tab Control")) -> ()
      }
      frame "Record Reason" {
        n112 = flat-sequence {
          frame #0 {
            n113 = local write "Tab Control"(T3."Recording Reason Sonde" ("Tab Control")) -> ()
          }
        }
      }
      frame "Continuous  Data" {
        n114 = local read "Found Quanta Sonde Com Port"() -> (w326:refnum<visa-resource-name>)
        n115 = control-ref of="Sonde Data Display"() -> (w330:refnum<vi>)
        n116 = local read "Sample Sheet Data Row Cluster 2"() -> (w322:T1)
        n117 = call "SDI-12 Continuous Operations.vi"("RS232 Port In"=w326, "Sensor Address In"="0", "Sonde Data Ctl Refnum"=w330, "Error In (No Error)"=w329) -> ("output cluster"=w327:T2, "Temperature"=w324:cluster{"Y":dbl[], "Y":dbl[]}[], "Sonde Data Display"=w323:T8, "Error Out"=w328:errorcluster)  [unwired: 8 in, 4 out]
        n118 = Bundle By Name(cluster=w322, "Sonde Data Cluster"=w327) -> (w325:T1)
        n119 = local write "Temperature"(w324) -> ()
        n120 = local write "Sonde Data Display"(w323) -> ()
        n121 = local write "Sample Sheet Data Row Cluster 2"(w325) -> ()
      }
      frame "Acq. Single Point" {
        n122 = invoke on="Record Single Sample" class="Bool" method="Reinit To Default"(error in=w345) -> (error out=w344:errorcluster)  [unwired: 2 in, 2 out]
        n123 = call <vilib>:"Clear Errors.vi"("error in (no error)"=w344) -> ("error out"=w332:errorcluster)  [unwired: 5 in, 1 out]
        n124 = call "get sample sheet data cells.vi"("error in (no error)"=w332, "NI_report in"=w363) -> ("error out"=w360:errorcluster, "data"=w362:string[][], "NI_report out"=w355:refnum<class "NI_report.lvclass">, "left edge output cluster"=w361:cluster{"row":i32, "column":i32})  [unwired: 5 in, 1 out]
        n125 = flat-sequence {
          tunnel: w360 -> [w423]
          tunnel: [w415] -> _
          tunnel: w361 -> [w421]
          tunnel: [w420] -> w359
          tunnel: [w419] -> _
          tunnel: [w418] -> w353
          tunnel: w362 -> [w415]
          frame #0 {
            n126 = Array Subset(array=w415, index (col)=2 ("index")) -> (w417:string[][])  [unwired: 3 in]
            n127 = local write "Sonde Data Array"(w417) -> ()
            n128 = local read "Current Sample Sheet"() -> (w414:string)
            n129 = call "find last occupied cell.vi"("data"=w415, "Active Sheet"=w414, "Header Rows to remove"=3, "sub array start"=w421, "error in (no error)"=w423) -> ("row max value"=w419:i32, 13:"start of last occupied row"=w418:cluster{"row":i32, "column":i32}, 14:"start of last occupied row"=→"last occupied cell's name":string, "error out"=w420:errorcluster)  [unwired: 4 in, 3 out]
            "row max value" <- w419
          }
        }
        n130 = local read "Found Quanta Sonde Com Port"() -> (w349:refnum<visa-resource-name>)
        n131 = Equal?(x=w349, y=refnum<visa-resource-name> refnum ("RS232 Port Out")) -> (x = y?=w351:bool)
        n132 = case shown="False" w351 {
          tunnel: w349 -> [w392 _]
          tunnel: [w383 w409] -> w352
          tunnel: w359 -> [w387 w412]
          tunnel: [w386 w412] -> w356
          tunnel: w339 -> [w382 w411]
          tunnel: [w381 w399] -> w338
          tunnel: [w380 w398] -> w337
          tunnel: w336 -> [w379 w410]
          tunnel: w335 -> [_ w395]
          frame False {
            n133 = control-ref of="Sonde Data Display"() -> (w388:refnum<vi>)
            n134 = local read "Sample Sheet Data Row Cluster 2"() -> (w384:T1)
            n135 = call "SDI-12 Single Operation with output cluster.vi"("RS232 Port In"=w392, "Sensor Address In"="0", "Sonde Data Ctl Refnum"=w388, "Error In (No Error)"=w387, "Time Array In"=w382, "Measurement Array In"=w379) -> ("time array out"=w381:dbl[], "Measurement  array Out"=w380:dbl[][], "output cluster"=w385:T2, "Temperature"=w390:cluster{"Y":dbl[], "Y":dbl[]}[], "Sonde Data Display"=w389:T8, "Error Out"=w386:errorcluster)  [unwired: 12 in, 4 out]
            n136 = local write "Temperature"(w390) -> ()
            n137 = local write "Sonde Data Display"(w389) -> ()
            n138 = Bundle By Name(cluster=w384, "Sonde Data Cluster"=w385) -> (w383:T1)
          }
          frame True {
            n139 = Get Date/Time In Seconds() -> (seconds since 1Jan1904=w401:timestamp)
            n140 = To Double Precision Float(number=w401) -> (double precision float=w400:dbl)
            n141 = Subtract(x=w400, y=w395) -> (x-y=w393:dbl)
            n142 = local read "Sample Sheet Data Row Cluster 2"() -> (w409:T1)
            n143 = local write "Current Time (s)"(w393) -> ()
            n144 = Unbundle By Name(w409) -> ("Sonde Data Cluster.Temp"=w394:dbl, "Sonde Data Cluster.pH"=w408:dbl, "Sonde Data Cluster.Specific\nConductance"=w407:dbl, "Sonde Data Cluster.Salinity"=w406:dbl, "Sonde Data Cluster.Dissolved\nOxygen"=w405:dbl, "Sonde Data Cluster.ORP"=w404:dbl)  [unwired: 1 out]
            n145 = Build Array(w394, w408, w407, w406, w405, 0.0 ("element"), w404) -> (w402:dbl[])
            n146 = Build Array (concatenate)(w411, w393) -> (w399:dbl[])
            n147 = Build Array (concatenate)(w410, w402) -> (w398:dbl[][])
            n148 = call "format into Sonde Vertical Graph Data Input.vi"("Sonde Measurement Array"=w398, "Time Array"=w399) -> ("Sonde Data Display"=w397:T8, "Temperature"=w396:cluster{"X":dbl[], "Y":dbl[]}[])  [unwired: 8 in]
            n149 = local write "Temperature"(w396) -> ()
            n150 = local write "Sonde Data Display"(w397) -> ()
          }
        }
        n151 = local write "Sample Sheet Data Row Cluster 2"(w352) -> ()
        n152 = call "write out sonde row.vi"("NI_report in"=w355, "Columns"=w358, "Column of Volume"=w357, "Sample Sheet Data Row Cluster"=w352, "row index"=w341, "error in (no error)"=w356, "start of last occupied row"=w353) -> ("NI_report out"=w347:refnum<class "NI_report.lvclass">, "row index out"=w340:i32, "error out"=w348:errorcluster)  [unwired: 6 in]
        n153 = flat-sequence {
          tunnel: w348 -> [w378]
          tunnel: w347 -> [w377]
          tunnel: [w376] -> w346
          tunnel: [w370] -> w343
          tunnel: [w368] -> w342
          frame #0 {
            (unwired) 3 ("Header Rows to remove")
            n154 = call <vilib>:"Clear Errors.vi"("error in (no error)"=w378) -> ("error out"=w364:errorcluster)  [unwired: 5 in, 1 out]
            n155 = local read "Current Sample Sheet"() -> (w366:string)
            n156 = call "get sample sheet data cells.vi"("error in (no error)"=w364, "NI_report in"=w377) -> ("error out"=w371:errorcluster, "data"=w372:string[][], "NI_report out"=w376:refnum<class "NI_report.lvclass">, "left edge output cluster"=w369:cluster{"row":i32, "column":i32})  [unwired: 5 in, 1 out]
            n157 = call "find last occupied cell.vi"("data"=w372, "Active Sheet"=w366, "Header Rows to remove"=3, "sub array start"=w369, "error in (no error)"=w371) -> ("row max value"=w367:i32, 13:"start of last occupied row"=w368:cluster{"row":i32, "column":i32}, 14:"start of last occupied row"=w365:string, "error out"=w370:errorcluster)  [unwired: 4 in, 3 out]
            n158 = Array Subset(array=w372, index (col)=2 ("index")) -> (w374:string[][])  [unwired: 3 in]
            n159 = local write "Sonde Data Array"(w374) -> ()
            n160 = local write "row max value"(w367) -> ()
            n161 = local write "last occupied cell's name"(w365) -> ()
          }
        }
      }
      frame "Write Sample Sheet" {
        n162 = Not Equal?(x=w445, y=w444) -> (x != y?=w443:bool)
        n163 = Decrement(x=w455) -> (x-1=w429:i32)
        n164 = case shown="True" w443 {
          tunnel: w456 -> [w459 w466]
          tunnel: w442 -> [_ w465]
          tunnel: w454 -> [w458 w464]
          tunnel: [w458 w463] -> w453
          tunnel: [w459 w462] -> w452
          tunnel: w447 -> [w457 w461]
          tunnel: [w457 w460] -> w446
          frame False {
          }
          frame True {
            n165 = flat-sequence {
              tunnel: [w475] -> w462
              tunnel: w466 -> [w474]
              tunnel: w465 -> [w471]
              tunnel: w464 -> [w470]
              tunnel: [w469] -> w463
              tunnel: w461 -> [w468]
              tunnel: [w467] -> w460
              frame #0 {
                n166 = Increment(x=w468) -> (x+1=w467:i32)
                n167 = call "write comment cell with column offset.vi"("Column Relative?"=TRUE, "comment string"="done", "error in (no error)"=w470, "start of last occupied row"=w471, "NI_report in"=w474) -> ("error out"=w469:errorcluster, "NI_report out"=w475:refnum<class "NI_report.lvclass">)  [unwired: 5 in]
              }
            }
          }
        }
        n168 = call "open select sample sheet.vi"("Number of Sample Sheets"=w448, "error in (no error)"=w453, "Worksheet Names"=w449, "Active Sample Sheet"=w446, "NI_report in"=w452) -> ("error out"=w439:errorcluster, "Current Sample Sheet"=w440:string, "NI_report out"=w438:refnum<class "NI_report.lvclass">)  [unwired: 3 in, 1 out]
        n169 = local write "Current Sample Sheet"(w440) -> ()
        n170 = local read "Current Sample Sheet"() -> (w431:string)
        n171 = call "get sample sheet data cells.vi"("error in (no error)"=w439, "NI_report in"=w438) -> ("error out"=w451:errorcluster, "data"=w436:string[][], "NI_report out"=w450:refnum<class "NI_report.lvclass">, "left edge output cluster"=w433:cluster{"row":i32, "column":i32})  [unwired: 5 in, 1 out]
        n172 = Array Subset(array=w436, index (col)=2 ("index")) -> (w434:string[][])  [unwired: 3 in]
        n173 = local write "Sonde Data Array"(w434) -> ()
        n174 = call "find last occupied cell.vi"("data"=w434, "Active Sheet"=w431, "Header Rows to remove"=3, "sub array start"=w433, "error in (no error)"=w451) -> ("row max value"=w432:i32, 13:"start of last occupied row"=w441:cluster{"row":i32, "column":i32}, 14:"start of last occupied row"=w430:string, "error out"=w424:errorcluster)  [unwired: 4 in, 3 out]
        n175 = local write "row max value"(w432) -> ()
        n176 = local write "last occupied cell's name"(w430) -> ()
      }
      frame "Init" {
        n177 = flat-sequence {
          tunnel: w479 -> [w509]
          tunnel: [w500] -> w477
          tunnel: [w495] -> w480
          frame #0 {
            n178 = call "create DAQ strings.vi"("error in (no error)"=w509, "MCC USB-DAQ Setup"="MCC USB-DAQ Setup") -> ("error IO"=w502:errorcluster, "Descriptions"=w498:string[], "delimited string"=w503:string, "Array"=w499:string[], "Voltage Range"=w508:dbl[])  [unwired: 5 in]
            "delimited string" <- w503
            "Active Channel Array" <- w499
            "Voltage Range" <- w508
            "Descriptions" <- w498
            n179 = call "Physical Channels to Number of channels.vi"("error in (no error)"=w502, "Physical Channel in"=w503) -> ("error out"=w504:errorcluster, "Number of Channels"=w506:i32)  [unwired: 7 in, 1 out]
            "Number of Channels" <- w506
            n180 = call "Calculate Rate from Num Channels and Max Rate.vi"("error in (no error)"=w504, "Channel Data Rate S/s"="Channel Data Rate S/s", "Number of Channels"=w506) -> ("error out"=w496:errorcluster, "Rate"=→"Rate":dbl)  [unwired: 7 in]
            n181 = for {
              tunnel: w499 -> [w516] mode=indexing
              tunnel: w508 -> [w515] mode=indexing
              tunnel: [w512] -> w495 mode=indexing
              shift-right: [w513] -> w501
              shift-left: w496 -> [w511]
              n182 = Negate(x=w515) -> (-x=w514:dbl)
              n183 = call-poly <vilib>:"ULx Create Virtual Channel.vi"("maximum value"=w515, "minimum value"=w514, "physical channels"=w516, "error in"=w511) -> ("task out"=w512:refnum<k24>, "error out"=w513:errorcluster)  [unwired: 10 in]
            }
            n184 = call "get 9V monitor voltage.vi"("error in (no error)"=w501, "Descriptions"=w498, "Array"=w499, "Array 2"=w495) -> ("error out"=w500:errorcluster, "9V Voltage Monitor"=→"9V Voltage Monitor":dbl)  [unwired: 6 in]
            "DAQ Error" <- w500
          }
        }
        n185 = flat-sequence {
          tunnel: w477 -> [w488]
          tunnel: [w488] -> w476
          frame #0 {
            w489 = T18."Enabled" ("Disabled")
            n186 = property on="Write Data to Spreadsheet" class="Bool"("DisabledEnum"=w489) -> (error out=w492:errorcluster)  [unwired: 2 in, 1 out]
            n187 = property on="Record Continuous Samples" class="Bool"(error in=w492, "DisabledEnum"=T18."Disabled and Grayed Out" ("Disabled")) -> (error out=w491:errorcluster)  [unwired: 1 in, 1 out]
            n188 = property on="Record Single Sample" class="Bool"(error in=w491, "DisabledEnum"=w489) -> (error out=w490:errorcluster)  [unwired: 1 in, 1 out]
            n189 = property on="Sample Not Collected" class="Bool"(error in=w490, "DisabledEnum"=w489) -> ()  [unwired: 1 in, 2 out]
            "Initialization Finished" <- TRUE
          }
        }
      }
      frame "Acq. DAQ data" {
        n190 = for {
          tunnel: w520 -> [w534] mode=indexing
          tunnel: w519 -> [w533]
          tunnel: [w531] -> w517 mode=indexing
          tunnel: [w530] -> _ mode=indexing
          tunnel: [w529] -> w518 mode=indexing
          n191 = call-poly <vilib>:"ULx Read.vi"("task in"=w534, "timeout"=10.0, "error in"=w533) -> ("task out"=w531:refnum<k24>, "data"=w529:dbl, "error out"=w530:errorcluster)  [unwired: 10 in]
        }
        "Raw Voltages" <- w518
      }
      frame "Exit" {
        n192 = case shown="No Error" w539 {
          tunnel: w535 -> [w575 _]
          tunnel: w539 -> [w574 w586]
          tunnel: [w573 w586] -> w537
          frame No Error {
            n193 = for {
              shift-right: [w577] -> w573
              shift-left: w574 -> [w578]
              tunnel: w575 -> [w576] mode=indexing
              n194 = while {
                shift-right: [w585] -> w580
                shift-left: w578 -> [w583]
                shift-right: [w584] -> w579
                shift-left: w576 -> [w582]
                stop <- w581 stop-if-true
                n195 = call <vilib>:"ULx Is Task Done.vi"("task in"=w582, "error in"=w583) -> ("task out"=w584:refnum<k24>, "task done?"=w581:bool, "error out"=w585:errorcluster)  [unwired: 11 in]
              }
              n196 = call <vilib>:"ULx Clear Task.vi"("task in"=w579, "error in"=w580) -> ("error out"=w577:errorcluster)  [unwired: 13 in]
            }
          }
          frame Error {
          }
        }
        n197 = local read "report file path"() -> (w552:path)
        n198 = flat-sequence {
          tunnel: [w592] -> w546
          tunnel: [w591] -> w549
          tunnel: w548 -> [w589]
          tunnel: w547 -> [w588]
          tunnel: w552 -> [w587]
          frame #0 {
            n199 = call-dynamic "Save Report to File.vi"("report in"=w588, "report file path"=w587, "prompt to replace? (F)"=FALSE, "error in (no error)"=w589) -> ("report out"=w592:refnum<class "NI_report.lvclass">, "error out"=w591:errorcluster)  [unwired: 10 in]
          }
        }
        n200 = call <userlib>:"Wait (ms)__ogtk.vi"("error in (no error)"=w549, "milliseconds to wait"=u32 5) -> ("error out"=w550:errorcluster)  [unwired: 8 in, 1 out]
        n201 = flat-sequence {
          tunnel: w550 -> [w561]
          tunnel: w546 -> [w559]
          tunnel: [w557] -> w540
          frame #0 {
            (unwired) FALSE ("Write Ini")
            n202 = call-dynamic "Dispose Report.vi"("report in"=w559, "save changes? (F)"=FALSE, "error in (no error)"=w561) -> ("error out"=w556:errorcluster)  [unwired: 12 in]
            n203 = case shown="False" "Save Configuration File?" {
              tunnel: [errorcluster {"status"=FALSE, "code"=0, "source"=""} ("error IO") w570] -> w558
              frame False {
              }
              frame True {
                n204 = local read "Config File Path"() -> (w569:path)
                n205 = call <vilib>:"Open Config Data.vi"("create file if necessary (T)"=TRUE ("Read Ini"), "configuration file path"=w569) -> ("error out"=w567:errorcluster, "refnum"=w564:T17)  [unwired: 7 in, 1 out]
                n206 = control-ref of="This VI"() -> (w563:refnum<vi>)
                n207 = call <userlib>:"Write Panel to INI__ogtk.vi"("error in (no error)"=w567, "VI ref"=w563, "refnum"=w564) -> ("error out"=w566:errorcluster, "refnum out"=w565:T17)  [unwired: 7 in]
                n208 = call <vilib>:"Clear Errors.vi"("error in (no error)"=w566) -> ("error out"=w572:errorcluster)  [unwired: 5 in, 1 out]
                n209 = call <vilib>:"Close Config Data.vi"("error in (no error)"=w572, "refnum"=w565) -> ("error out"=w571:errorcluster)  [unwired: 8 in, 1 out]
                n210 = Merge Errors(w571, w566) -> (w570:errorcluster)
              }
            }
            n211 = Merge Errors(w558, w556) -> (w557:errorcluster)
          }
        }
        n212 = flat-sequence {
          tunnel: [TRUE ("aborted?")] -> w538
          tunnel: [w553] -> w536
          tunnel: w537 -> [w553]
          frame #0 {
          }
        }
      }
    }
    "Stop 2" <- w246
    "consumer loop" <- w275
  }
  "Feet of\nStainless to be\nUsed (Count)" <- w2
  "Feet of Stainless 2" <- w1
  n213 = Merge Errors(w29, w28) -> (→"error out":errorcluster)
